vi "Set UUT Serial Port Parameters.vi"(0 "VISA resource name":refnum<visa-resource-name>, 1 "Baud Rate (9600)":u32=9600, 5 "Flow Control (0: Xon/Xoff)":u32(ring) items=["Xon/Xoff", "None", "Rts/Cts"], 7 "Number Data Bits (1: 8 bits)":u32(ring)=1 items=["7 bits", "8 bits"], 9 "Number Stop Bits (0: 1 bit)":u32(ring) items=["1 bit", "2 bits"], 11 "error in (no error)":errorcluster, 12 "Parity  (0: None)":u32(ring) items=["None", "Odd", "Even"]) -> (4 "VISA resource name out":refnum<visa-resource-name>, 15 "error out":errorcluster)   [LabVIEW 2014, in "Fluke 5XXX Series Multicalibrators.lvlib"]
doc: "This VI Sets the RS-232-C settings for the Calibrator rear panel SERIAL 2 TO UUT serial port, which is saved in the Calibrator non-volatile memory. (While saving configuration data in the non-volatile memory, a period of about 2 seconds, the Calibrator does not respond to remote commands.)\n\nNote:\n\nThis VI is available only for instrument models 5500A and 5520A."
uses:
  Fluke 5XXX Series Multicalibrators.lvlib
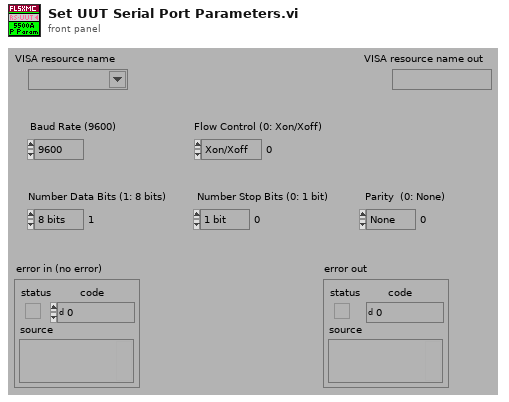
[diagram p1: front panel]
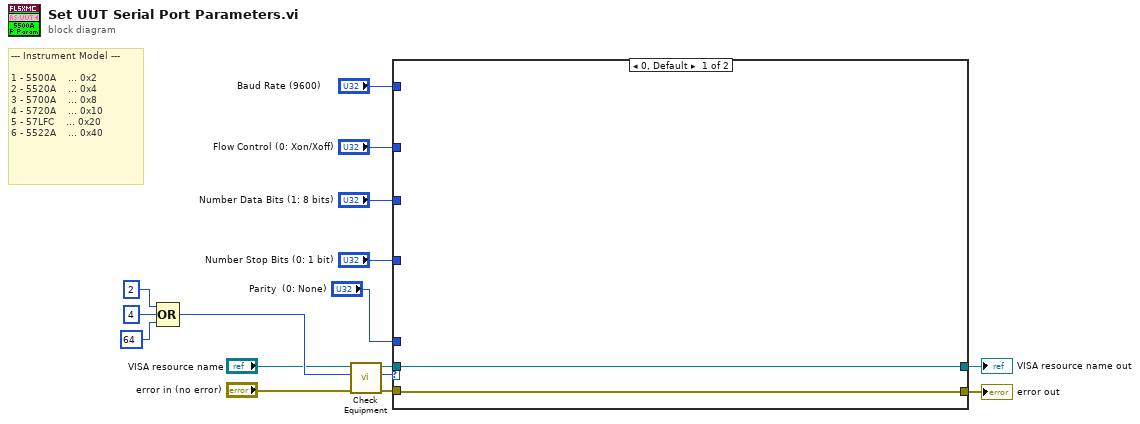
[diagram p0: block diagram]
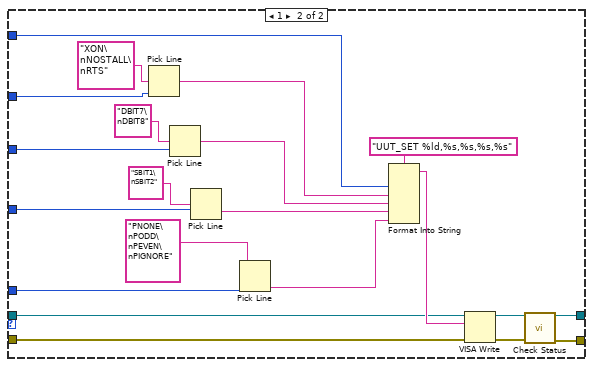
[diagram p2: hidden frame]
diagram:
  # "--- Instrument Model ---\n\n1 - 5500A    ... 0x2\n2 - 5520A    ... 0x4\n3 - 5700A    ... 0x8\n4 - 5720A    ... 0x10\n5 - 57LFC    ... 0x20\n6 - 5522A    ... 0x40"
  n1 = Compound Arithmetic op=OR(2 ("Numeric"), 4 ("Numeric"), 64 ("Numeric")) -> (w7:i32)
  n2 = call "Check Equipment.vi"("error in (no error)"="error in (no error)", "Bit Mask"=w7, "VISA resource name"="VISA resource name") -> ("error out"=w2:errorcluster, "Present?"=w3:u32, "VISA resource name out"=w4:refnum<visa-resource-name>)  [unwired: 6 in]
  n3 = case shown="0, Default" w3 {
    tunnel: "Baud Rate (9600)" -> [_ w20]
    tunnel: [w17 w30] -> w15
    tunnel: w4 -> [w18 w29]
    tunnel: "Flow Control (0: Xon/Xoff)" -> [_ w28]
    tunnel: "Number Data Bits (1: 8 bits)" -> [_ w27]
    tunnel: "Number Stop Bits (0: 1 bit)" -> [_ w26]
    tunnel: "Parity  (0: None)" -> [_ w25]
    tunnel: [w18 w21] -> w10
    tunnel: w2 -> [w17 w19]
    frame 0, Default {
    }
    frame 1 {
      n4 = Pick Line(multi-line string="XON\nNOSTALL\nRTS" ("Reset Command"), line index=w28) -> (output string=w35:string)  [unwired: 1 in]
      n5 = Pick Line(multi-line string="DBIT7\nDBIT8" ("Reset Command"), line index=w27) -> (output string=w22:string)  [unwired: 1 in]
      n6 = Pick Line(multi-line string="SBIT1\nSBIT2" ("Reset Command"), line index=w26) -> (output string=w23:string)  [unwired: 1 in]
      n7 = Pick Line(multi-line string="PNONE\nPODD\nPEVEN\nPIGNORE" ("Reset Command"), line index=w25) -> (output string=w24:string)  [unwired: 1 in]
      n8 = Format Into String(format string="UUT_SET %ld,%s,%s,%s,%s" ("Reset Command"), w20, w35, w22, w23, w24) -> (resulting string=w36:string)  [unwired: 2 in, 1 out]
      n9 = VISA Write(VISA resource name=w29, write buffer=w36, error in (no error)=w19) -> (VISA resource name out=w39:refnum<visa-resource-name>, error out=w38:errorcluster)  [unwired: 1 out]
      n10 = call "Check Status.vi"("VISA resource name"=w39, "error in (no error)"=w38) -> ("VISA resource name out"=w21:refnum<visa-resource-name>, "error out"=w30:errorcluster)  [unwired: 12 in]
    }
  }
  "VISA resource name out" <- w10
  "error out" <- w15
